vi "Data_Aquisition_cRIO3.vi"() -> ()   [LabVIEW 2016]
uses:
  <vilib>/Platform/TimedLoop/XDataNode/timing_clust.ctl
  <vilib>/Platform/TimedLoop/XDataNode/nitl_modes.ctl
  <vilib>/Platform/TimedLoop/XDataNode/wakeup.ctl
  <vilib>/Utility/file.llb/Write Delimited Spreadsheet (string).vi
  <vilib>/Platform/TimedLoop/XDataNode/loadnilvce.vi
  <vilib>/Utility/file.llb/Write Delimited Spreadsheet (DBL).vi
  <vilib>/Platform/TimedLoop/XDataNode/XDataNode.xnode
  <vilib>/Platform/TimedLoop/XDataNode/XDNodeRunTimeDep.lvlib
panel:
  in  "Mod 2 Labels":string[][](array[string])
  in  "Mod 1 Labels":string[][](array[string])
  in  "Mod 4 Labels":string[][](array[string])
  in  "Mod 3 Labels":string[][](array[string])
  out "data":dbl[][](array[numeric])
  out "headers":string[][](array[string])
  out "Time":string="113841.85"
  out "Date":string="09142017"
  in  "Buffer Size":i32=100
  out "Saving?":bool=TRUE
  out "new file path (Not A Path if cancelled)":path=path "u:/_09142017_113831.csv"
  in  "File Name:":string
  out "error out":errorcluster
  out "iter number":i32=236
  in  "stop":bool
  in  "error in":errorcluster
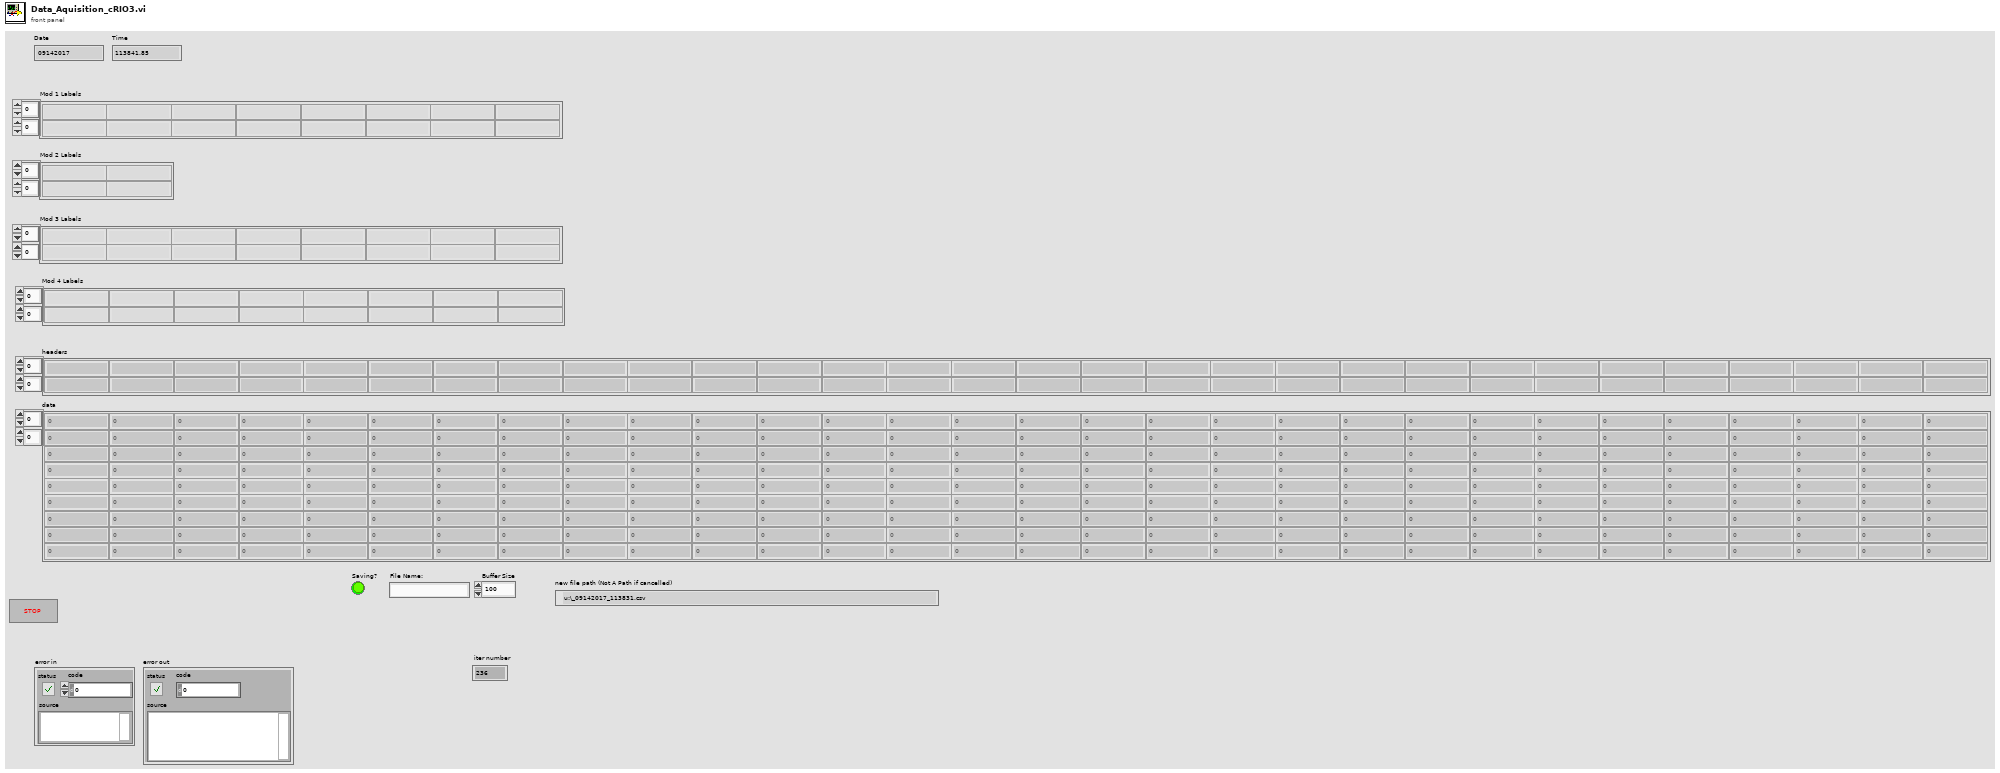
[diagram p1: front panel]
types:
  T1 = typedef "XDNodeRunTimeDep.lvlib/timing_clust.ctl" = cluster{"Expected End [f-1]":u64, "Actual End [f-1]":u64, "Finished Late? [f-1]":bool, "Expected End [i-1]":u64, "Actual End [i-1]":u64, "Finished Late? [i-1]":bool, "Expected Start [i]":u64, "Actual Start [i]":u64, "Expected Start [f]":u64, "Actual Start [f]":u64, "Source Name":string, "Structure Name":string, "Period":i64, "Deadline":i64, "Offset":i64, "Start":i64, "Priority":i32, "Timeout":i32, "Mode":T2, "Wakeup Reason":T3, "Error":errorcluster, "Source Type":string, "Secondary Source Type":string, "Global End Time":u64, "Global Start Time":u64, "Frame Duration":u64, "Iteration Duration":u64, "Assigned CPU":i32, "I/O Scan Engine Mode":u32}
  T2 = typedef "XDNodeRunTimeDep.lvlib/nitl_modes.ctl" = enum32{"No Change", "Process missed periods, maintain original phase", "Discard missed periods, maintain original phase", "Process missed periods, ignore original phase", "Discard missed periods, ignore original phase"}
  T3 = typedef "XDNodeRunTimeDep.lvlib/wakeup.ctl" = enum32{"Normal", "Aborted", "Asynchronous wakeup", "Timing source error", "Timed loop error", "Timeout"}
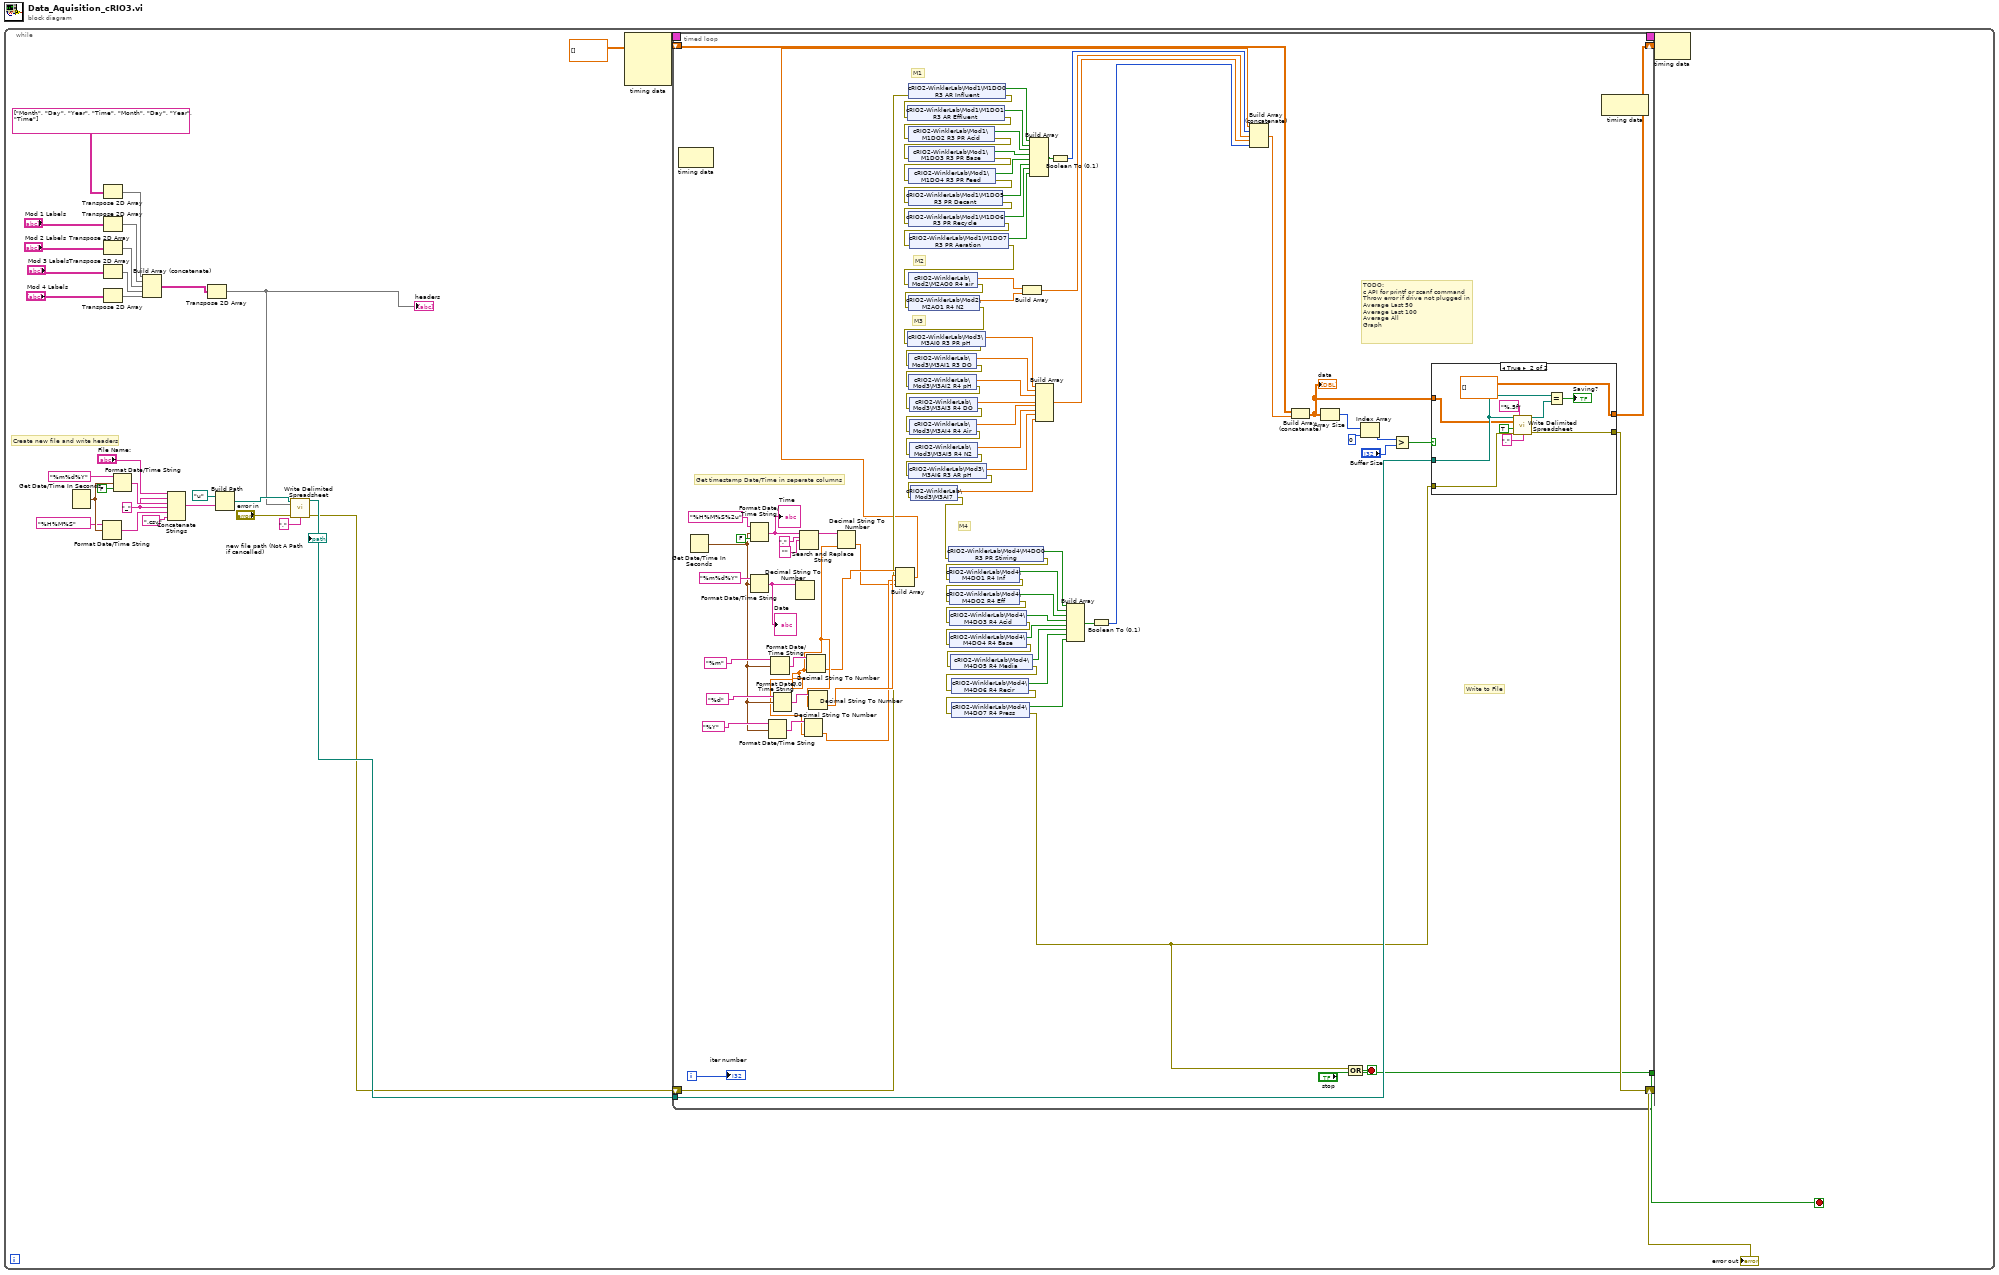
[diagram p0: block diagram]
diagram:
  n1 = while {
    stop <- w18 stop-if-true
    w21 = "_" ("string")
    # "Create new file and write headers"
    n2 = Get Date/Time In Seconds() -> (seconds since 1Jan1904=w26:timestamp)
    n3 = Format Date/Time String(time format string (%c)="%H%M%S", seconds (now)=w26) -> (date/time string=w20:string)  [unwired: 1 in]
    n4 = Transpose 2D Array(2D array=string[][] [["Month", "Day", "Year", "Time"], ["Month", "Day", "Year", "Time"]]) -> (transposed array=w10:string[][])
    n5 = Transpose 2D Array(2D array="Mod 1 Labels") -> (transposed array=w9:string[][])
    n6 = Transpose 2D Array(2D array="Mod 2 Labels") -> (transposed array=w8:string[][])
    n7 = Transpose 2D Array(2D array="Mod 3 Labels") -> (transposed array=w7:string[][])
    n8 = Transpose 2D Array(2D array="Mod 4 Labels") -> (transposed array=w6:string[][])
    n9 = Format Date/Time String(time format string (%c)="%m%d%Y", seconds (now)=w26, UTC format=FALSE) -> (date/time string=w22:string)
    n10 = Build Array (concatenate)(w10, w9, w8, w7, w6) -> (w12:string[][])
    n11 = Concatenate Strings("File Name:", w21, w22, w21, w20, ".csv" ("string")) -> (w19:string)
    n12 = Transpose 2D Array(2D array=w12) -> (transposed array=w5:string[][])
    "headers" <- w5
    n13 = Build Path(base path=path "u:/" ("Save to:"), name or relative path=w19) -> (appended path=w29:path)
    n14 = call-poly <vilib>:"Write Delimited Spreadsheet.vi"("file path (dialog if empty)"=w29, "2D data"=w5, "error in (no error)"="error in", "delimiter (\\t)"="," ("delimiter (\\t)")) -> ("new file path (Not A Path if cancelled)"=w33:path, "error out"=w32:errorcluster)  [unwired: 10 in]
    "new file path (Not A Path if cancelled)" <- w33
    n15 = node-c288() -> (w17:T1)  [unwired: 4 in]
    n16 = timed-loop {
      tunnel: w33 -> [w120]
      shift-right: [w106] -> _
      shift-left: dbl[][] [] -> [w125]
      shift-right: [w118] -> w13
      shift-left: w32 -> [w85]
      tunnel: ["stop"] -> w18
      timing: w17 -> [_]
      timing-out: [_] -> w16
      i -> [w126]
      stop <- w127 stop-if-true
      w97 = 0.0
      # "M4"
      # "M3"
      # "M2"
      # "M1"
      # "TODO: \nc API for printf or scanf command\nThrow error if drive not plugged in\nAverage Last 50\nAverage Last 100\nAverage All\nGraph"
      # "Write to File"
      # "Get timestamp Date/Time in seperate columns"
      n17 = node-c288() -> ()  [unwired: 1 in, 1 out]
      n18 = Get Date/Time In Seconds() -> (seconds since 1Jan1904=w98:timestamp)
      n19 = Format Date/Time String(time format string (%c)="%H%M%S%2u", seconds (now)=w98, UTC format=FALSE) -> (date/time string=w113:string)
      "Time" <- w113
      n20 = Format Date/Time String(time format string (%c)="%m%d%Y", seconds (now)=w98) -> (date/time string=w110:string)  [unwired: 1 in]
      "Date" <- w110
      n21 = Format Date/Time String(time format string (%c)="%Y", seconds (now)=w98) -> (date/time string=w99:string)  [unwired: 1 in]
      n22 = Format Date/Time String(time format string (%c)="%m", seconds (now)=w98) -> (date/time string=w103:string)  [unwired: 1 in]
      n23 = Format Date/Time String(time format string (%c)="%d", seconds (now)=w98) -> (date/time string=w101:string)  [unwired: 1 in]
      n24 = Decimal String To Number(string=w110) -> ()  [unwired: 2 in, 2 out]
      n25 = Search and Replace String(input string=w113, search string=".", replace string="") -> (result string=w112:string)  [unwired: 5 in, 3 out]
      n26 = Decimal String To Number(string=w99, default (0L)=w97) -> (number=w94:dbl)  [unwired: 1 in, 1 out]
      n27 = Decimal String To Number(string=w103, default (0L)=w97) -> (number=w96:dbl)  [unwired: 1 in, 1 out]
      n28 = Decimal String To Number(string=w101, default (0L)=w97) -> (number=w95:dbl)  [unwired: 1 in, 1 out]
      n29 = Decimal String To Number(string=w112, default (0L)=w97) -> (number=w93:dbl)  [unwired: 1 in, 1 out]
      n30 = Build Array(w96, w95, w94, w93) -> (w69:dbl[])
      n31 = shared-variable "cRIO2-WinklerLab\\Mod1\\M1DO0 R3 AR Influent"(error in=w85) -> (w84:bool, error out=w92:errorcluster)
      n32 = shared-variable "cRIO2-WinklerLab\\Mod1\\M1DO1 R3 AR Effluent"(error in=w92) -> (w83:bool, error out=w91:errorcluster)
      n33 = shared-variable "cRIO2-WinklerLab\\Mod1\\M1DO2 R3 PR Acid"(error in=w91) -> (w82:bool, error out=w90:errorcluster)
      n34 = shared-variable "cRIO2-WinklerLab\\Mod1\\M1DO3 R3 PR Base"(error in=w90) -> (w81:bool, error out=w89:errorcluster)
      n35 = shared-variable "cRIO2-WinklerLab\\Mod1\\M1DO4 R3 PR Feed"(error in=w89) -> (w80:bool, error out=w88:errorcluster)
      n36 = shared-variable "cRIO2-WinklerLab\\Mod1\\M1DO5 R3 PR Decant"(error in=w88) -> (w79:bool, error out=w87:errorcluster)
      n37 = shared-variable "cRIO2-WinklerLab\\Mod1\\M1DO6 R3 PR Recycle"(error in=w87) -> (w78:bool, error out=w86:errorcluster)
      n38 = shared-variable "cRIO2-WinklerLab\\Mod1\\M1DO7 R3 PR Aeration"(error in=w86) -> (w77:bool, error out=w75:errorcluster)
      n39 = shared-variable "cRIO2-WinklerLab\\Mod2\\M2AO0 R4 air"(error in=w75) -> (w74:dbl, error out=w76:errorcluster)
      n40 = shared-variable "cRIO2-WinklerLab\\Mod2\\M2AO1 R4 N2"(error in=w76) -> (w73:dbl, error out=w63:errorcluster)
      n41 = shared-variable "cRIO2-WinklerLab\\Mod3\\M3AI0 R3 PR pH"(error in=w63) -> (w62:dbl, error out=w68:errorcluster)
      n42 = shared-variable "cRIO2-WinklerLab\\Mod3\\M3AI1 R3 DO"(error in=w68) -> (w61:dbl, error out=w67:errorcluster)
      n43 = shared-variable "cRIO2-WinklerLab\\Mod3\\M3AI2 R4 pH"(error in=w67) -> (w60:dbl, error out=w66:errorcluster)
      n44 = shared-variable "cRIO2-WinklerLab\\Mod3\\M3AI3 R4 DO"(error in=w66) -> (w59:dbl, error out=w65:errorcluster)
      n45 = shared-variable "cRIO2-WinklerLab\\Mod3\\M3AI4 R4 Air"(error in=w65) -> (w58:dbl, error out=w64:errorcluster)
      n46 = shared-variable "cRIO2-WinklerLab\\Mod3\\M3AI5 R4 N2"(error in=w64) -> (w57:dbl, error out=w38:errorcluster)
      n47 = shared-variable "cRIO2-WinklerLab\\Mod3\\M3AI6 R3 AR pH"(error in=w38) -> (w37:dbl, error out=w36:errorcluster)
      n48 = shared-variable "cRIO2-WinklerLab\\Mod3\\M3AI7"(error in=w36) -> (w35:dbl, error out=w34:errorcluster)
      n49 = shared-variable "cRIO2-WinklerLab\\Mod4\\M4DO0 R3 PR Stirring"(error in=w34) -> (w54:bool, error out=w45:errorcluster)
      n50 = shared-variable "cRIO2-WinklerLab\\Mod4\\M4DO1 R4 Inf"(error in=w45) -> (w53:bool, error out=w44:errorcluster)
      n51 = shared-variable "cRIO2-WinklerLab\\Mod4\\M4DO2 R4 Eff"(error in=w44) -> (w47:bool, error out=w43:errorcluster)
      n52 = shared-variable "cRIO2-WinklerLab\\Mod4\\M4DO3 R4 Acid"(error in=w43) -> (w48:bool, error out=w42:errorcluster)
      n53 = shared-variable "cRIO2-WinklerLab\\Mod4\\M4DO4 R4 Base"(error in=w42) -> (w49:bool, error out=w41:errorcluster)
      n54 = shared-variable "cRIO2-WinklerLab\\Mod4\\M4DO5 R4 Media"(error in=w41) -> (w50:bool, error out=w40:errorcluster)
      n55 = shared-variable "cRIO2-WinklerLab\\Mod4\\M4DO6 R4 Recir"(error in=w40) -> (w51:bool, error out=w39:errorcluster)
      n56 = shared-variable "cRIO2-WinklerLab\\Mod4\\M4DO7 R4 Press"(error in=w39) -> (w52:bool, error out=w56:errorcluster)
      n57 = Build Array(w74, w73) -> (w71:dbl[])
      n58 = Build Array(w84, w83, w82, w81, w80, w79, w78, w77) -> (w72:bool[])
      n59 = Build Array(w62, w61, w60, w59, w58, w57, w37, w35) -> (w108:dbl[])
      n60 = Boolean To (0,1)(Boolean=w72) -> (0, 1=w70:i16[])
      n61 = Build Array(w54, w53, w47, w48, w49, w50, w51, w52) -> (w46:bool[])
      n62 = Boolean To (0,1)(Boolean=w46) -> (0, 1=w55:i16[])
      n63 = Build Array (concatenate)(w69, w70, w71, w108, w55) -> (w107:dbl[])
      n64 = Build Array (concatenate)(w125, w107) -> (w105:dbl[][])
      "data" <- w105
      n65 = Array Size(array=w105) -> (size(s)=w124:i32[])
      n66 = Compound Arithmetic op=OR(w56, "stop") -> (w127:bool)
      n67 = Index Array(array=w124, index=0) -> (element=w122:i32)
      n68 = Greater?(x=w122, y="Buffer Size") -> (0:w121:bool)
      n69 = case shown="True" w121 {
        tunnel: w105 -> [w131 w132]
        tunnel: w120 -> [_ w139]
        tunnel: [w131 dbl[][] []] -> w106
        tunnel: [w130 w138] -> w118
        tunnel: w56 -> [w130 w133]
        frame False {
        }
        frame True {
          n70 = call-poly <vilib>:"Write Delimited Spreadsheet.vi"("file path (dialog if empty)"=w139, "format (%.3f)"="%.5f", "2D data"=w132, "append to file? (new file:F)"=TRUE, "error in (no error)"=w133, "delimiter (\\t)"="," ("delimiter (\\t)")) -> ("new file path (Not A Path if cancelled)"=w140:path, "error out"=w138:errorcluster)  [unwired: 8 in]
          n71 = Equal?(x=w139, y=w140) -> (x = y?=→"Saving?":bool)
        }
      }
      n72 = node-c288() -> ()  [unwired: 1 in, 1 out]
      "iter number" <- w126
    }
    "error out" <- w13
    n73 = node-c288(w16) -> ()  [unwired: 1 out]
  }
